vi "Send_SET_1BIT.vi"(8 "error in (no error)":errorcluster, 9 "Encender?":bool, 10 "Channel":u8, 11 "NXP in":refnum<class "NXP.lvclass">) -> (0 "error out":errorcluster, 2 "buffer":string, 3 "NXP out":refnum<class "NXP.lvclass">)   [LabVIEW 2019, in "NXP.lvclass"]
uses:
  NXP.lvclass
  Clase Padre/Serial Device.lvclass
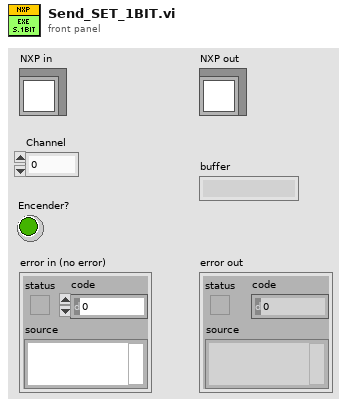
[diagram p1: front panel]
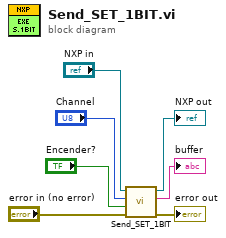
[diagram p0: block diagram]
diagram:
  n1 = call-parent "Send_SET_1BIT.vi"("error in (no error)"="error in (no error)", "Encender?"="Encender?", "Channel"="Channel", "Serial Device in"="NXP in") -> ("error out"=→"error out":errorcluster, "buffer"=→"buffer":string, "Serial Device out"=→"NXP out":refnum<class "NXP.lvclass">)  [unwired: 5 in]
